vi "CameraSetup.vi"(8 "error in (no error)":errorcluster, 10 "Task":T1(ring), 11 "SRV In":refnum<k5>) -> (0 "error out":errorcluster, 3 "SRV Out":refnum<k5>)   [LabVIEW 2014]
doc: "Modified for Benilde St. Margaret's School - Tim Jump\nBy Doug Schmertman - Logic PD\nCopyright 2012"
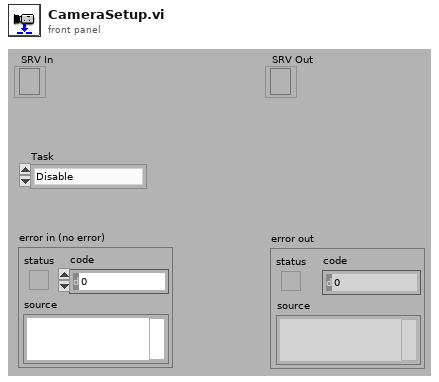
[diagram p1: front panel]
types:
  T1 = enum16{"Disable", "Frame Differencing", "Color Segmentation", "Edge Detection", "Horizon detection", "Obstacle detection", "Stereo processing"}
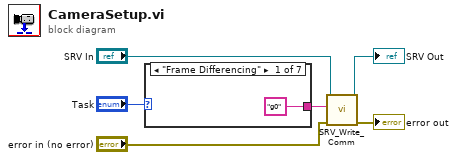
[diagram p0: block diagram]
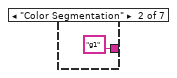
[diagram p2: hidden frame]
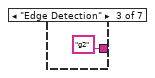
[diagram p3: hidden frame]
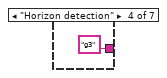
[diagram p4: hidden frame]
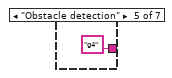
[diagram p5: hidden frame]
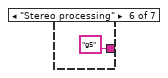
[diagram p6: hidden frame]
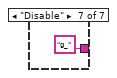
[diagram p7: hidden frame]
diagram:
  n1 = case shown="\"Frame Differencing\"" "Task" {
    tunnel: ["g0" ("Command Sent") "g1" ("Command Sent") "g2" ("Command Sent") "g3" ("Command Sent") "g4" ("Command Sent") "g5" ("Command Sent") "g_" ("Command Sent")] -> w6
    frame "Frame Differencing" {
    }
    frame "Color Segmentation" {
    }
    frame "Edge Detection" {
    }
    frame "Horizon detection" {
    }
    frame "Obstacle detection" {
    }
    frame "Stereo processing" {
    }
    frame "Disable" {
    }
  }
  n2 = call "SRV_Write_Comm.vi"("error in (no error)"="error in (no error)", "Command Sent"=w6, "SRV In"="SRV In") -> ("error out"=→"error out":errorcluster, "SRV Out"=→"SRV Out":refnum<k5>)  [unwired: 6 in, 1 out]
